vi "Post-Build Action - Remove C Dir.vi"(5 "Files Generated by Build":path[](array[path]), 6 "Top Level/Always Included VIs":path[](array[path]), 7 "Destination Path":path, 8 "error in (no error)":errorcluster, 9 "Target Name":string, 10 "Build Specification Name":string, 11 "Project Path":path) -> (0 "error out":errorcluster)   [LabVIEW 2011]
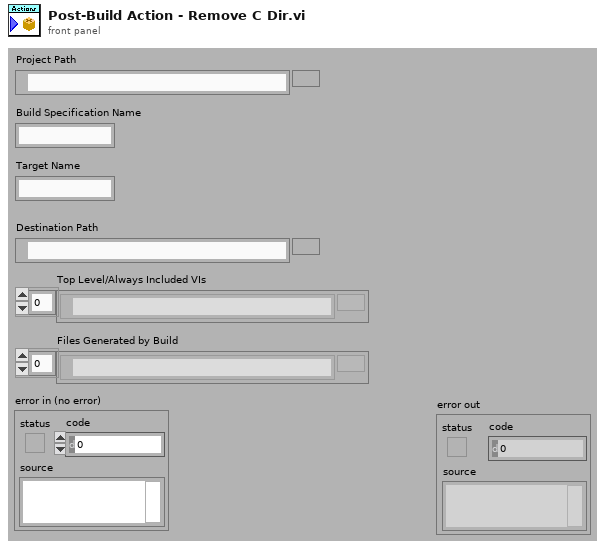
[diagram p1: front panel]
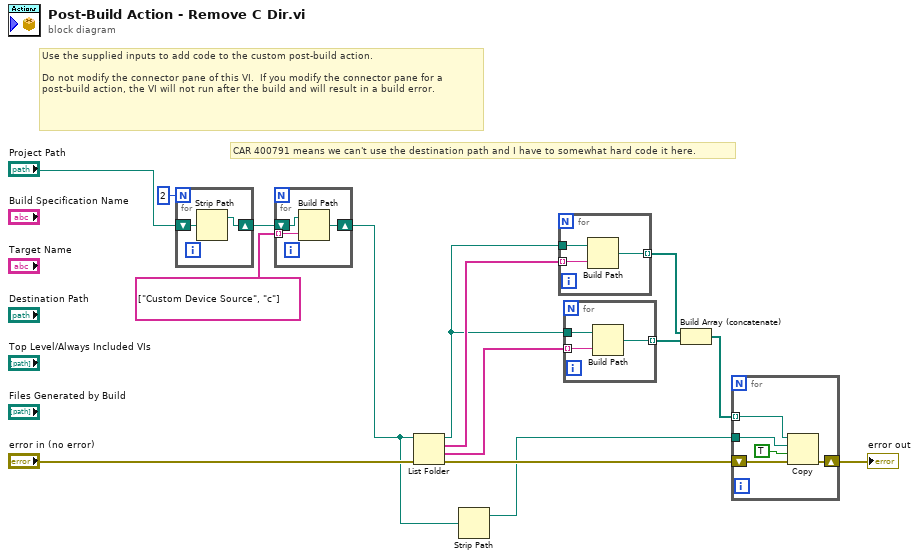
[diagram p0: block diagram]
diagram:
  # "CAR 400791 means we can't use the destination path and I have to somewhat hard code it here."
  # "Use the supplied inputs to add code to the custom post-build action.\n\nDo not modify the connector pane of this VI.  If you modify the connector pane for a post-build action, the VI will not run after the build and will result in a build error."
  n1 = for {
    N: 2 -> [_]
    shift-right: [w16] -> w3
    shift-left: "Project Path" -> [w17]
    n2 = Strip Path(path=w17) -> (stripped path=w16:path)  [unwired: 1 out]
  }
  n3 = for {
    shift-right: [w20] -> w1
    shift-left: w3 -> [w19]
    tunnel: string[] ["Custom Device Source", "c"] -> [w18] mode=indexing
    n4 = Build Path(base path=w19, name or relative path=w18) -> (appended path=w20:path)
  }
  n5 = List Folder(path=w1, error in="error in (no error)") -> (path out=w11:path, filenames=w15:string[], folder names=w12:string[], error out=w9:errorcluster)  [unwired: 2 in]
  n6 = Strip Path(path=w1) -> (stripped path=w7:path)  [unwired: 1 out]
  n7 = for {
    tunnel: w15 -> [w22] mode=indexing
    tunnel: w11 -> [w23]
    tunnel: [w21] -> w14 mode=indexing
    n8 = Build Path(base path=w23, name or relative path=w22) -> (appended path=w21:path)
  }
  n9 = for {
    tunnel: w12 -> [w25] mode=indexing
    tunnel: w11 -> [w26]
    tunnel: [w24] -> w10 mode=indexing
    n10 = Build Path(base path=w26, name or relative path=w25) -> (appended path=w24:path)
  }
  n11 = Build Array (concatenate)(w14, w10) -> (w13:path[])
  n12 = for {
    tunnel: w13 -> [w28] mode=indexing
    shift-right: [w29] -> w6
    shift-left: w9 -> [w30]
    tunnel: w7 -> [w27]
    n13 = Copy(8:w30, 9:TRUE ("overwrite (F)"), 10:w27, 11:w28) -> (0:w29:errorcluster)  [unwired: 1 in, 2 out]
  }
  "error out" <- w6
